vi "2_color_temp_subVI.vi"(8 "E1 2":dbl[](array[numeric]), 9 "E1":dbl[](array[numeric]), 10 "In_WL1 2":dbl[](array[numeric]), 11 "In_WL1":dbl[](array[numeric])) -> (3 "FT":dbl[](array[numeric]))   [LabVIEW 2017]
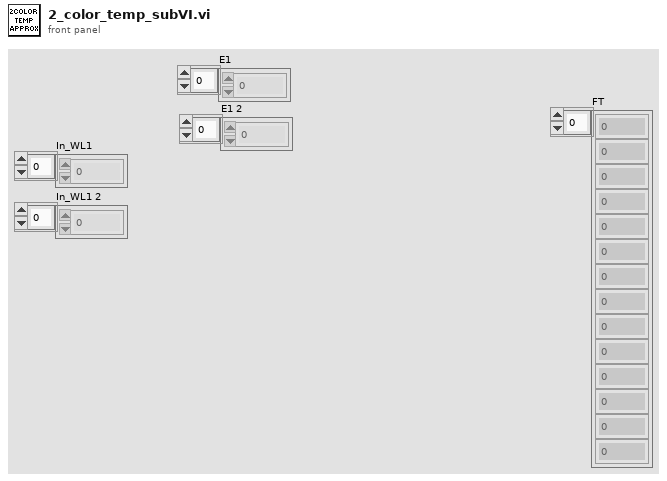
[diagram p1: front panel]
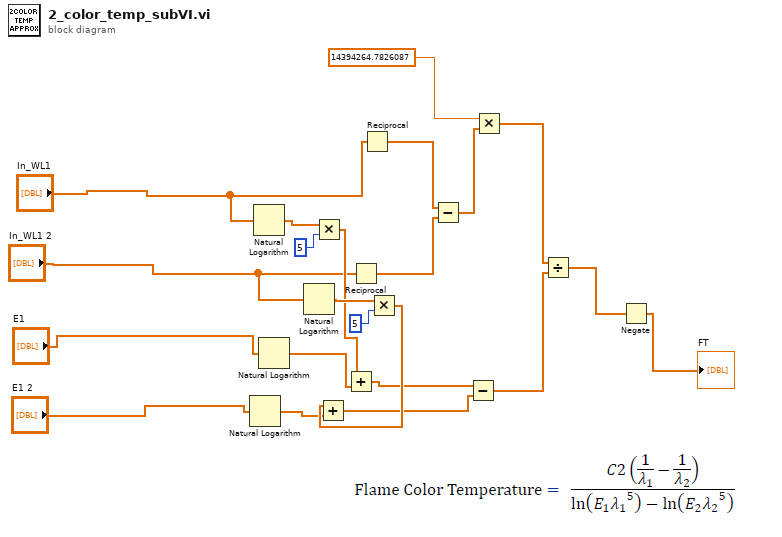
[diagram p0: block diagram]
diagram:
  n1 = Natural Logarithm(1:"E1 2") -> (0:w11:dbl[])
  n2 = Natural Logarithm(1:"In_WL1") -> (0:w16:dbl[])
  n3 = Natural Logarithm(1:"E1") -> (0:w18:dbl[])
  n4 = Natural Logarithm(1:"In_WL1 2") -> (0:w14:dbl[])
  n5 = Multiply(x=w16, y=5) -> (x*y=w13:dbl[])
  n6 = Add(x=w13, y=w18) -> (x+y=w10:dbl[])
  n7 = Reciprocal(x="In_WL1 2") -> (1/x=w20:dbl[])
  n8 = Reciprocal(x="In_WL1") -> (1/x=w21:dbl[])
  n9 = Multiply(x=w14, y=5) -> (x*y=w12:dbl[])
  n10 = Add(x=w12, y=w11) -> (x+y=w9:dbl[])
  n11 = Subtract(x=w21, y=w20) -> (x-y=w19:dbl[])
  n12 = Subtract(x=w10, y=w9) -> (x-y=w7:dbl[])
  n13 = Multiply(x=14394264.7826087, y=w19) -> (x*y=w8:dbl[])
  n14 = Divide(x=w8, y=w7) -> (x/y=w2:dbl[])
  n15 = Negate(x=w2) -> (-x=→"FT":dbl[])
